vi "GetPeakPosition.vi"(11 "Input cluster":cluster{dbl[], dbl[]}) -> (3 "Peak position [mm]":dbl)   [LabVIEW 2013]
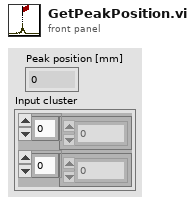
[diagram p1: front panel]
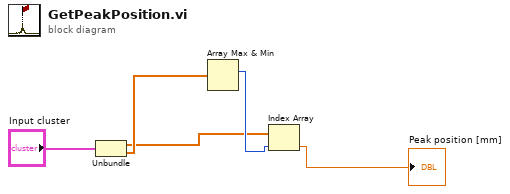
[diagram p0: block diagram]
diagram:
  n1 = Unbundle("Input cluster") -> (w2:dbl[], w4:dbl[])
  n2 = Array Max & Min(array=w4) -> (max index (indices)=w3:i32)  [unwired: 3 out]
  n3 = Index Array(array=w2, index=w3) -> (element=→"Peak position [mm]":dbl)
